vi "receive.vi"(8 "error in (no error)":errorcluster, 11 "ILCCommunications in":refnum<class "ILCCommunications.lvclass">) -> (0 "error out":errorcluster, 3 "ILCCommunications out":refnum<class "ILCCommunications.lvclass">)   [LabVIEW 2016, in "ILCCommunications.lvclass"]
uses:
  ILCCommunications.lvclass
  ILCCommunications.lvclass/ILCCommunications.ctl
  Common_RT_Modbus/DynamicFrameParser/DynamicFrameParser.lvclass
  Common_RT_FPGA/IReadU16FIFO/IReadU16FIFO.lvclass
  Common_RT_Modbus/IModbus/IModbus.lvclass
  Common_RT_HPILC/HPILC/HPILC.lvclass
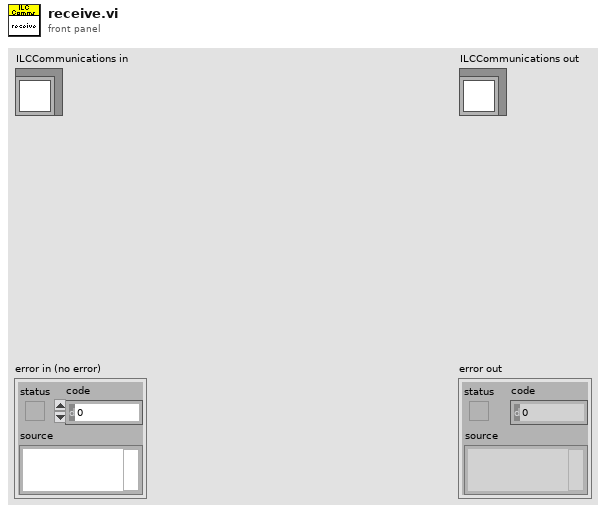
[diagram p1: front panel]
types:
  T1 = typedef "RTModbus.lvlib/RxFrame.ctl" = cluster{"Data":u8[], "Timestamp":u64}
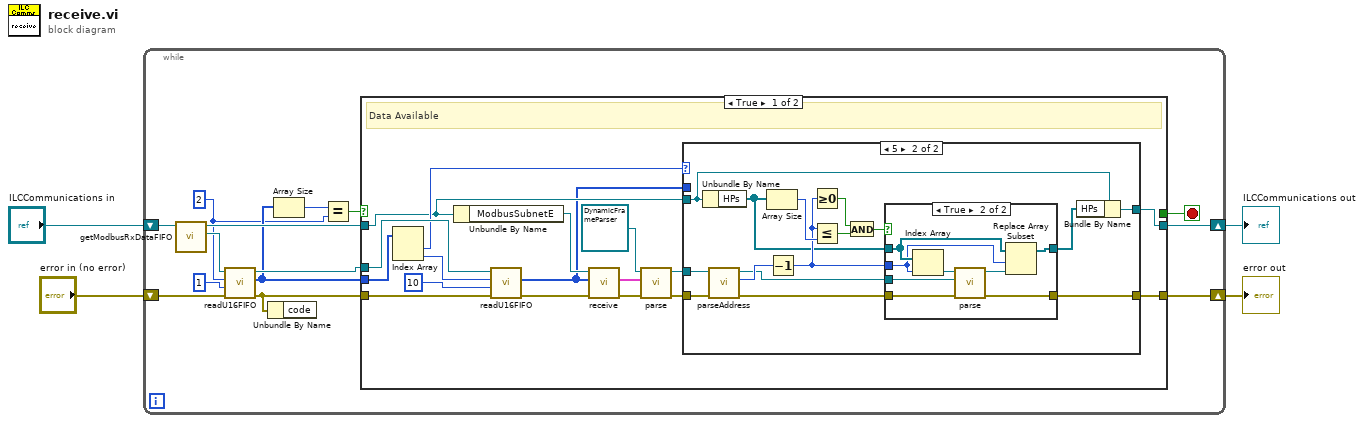
[diagram p0: block diagram]
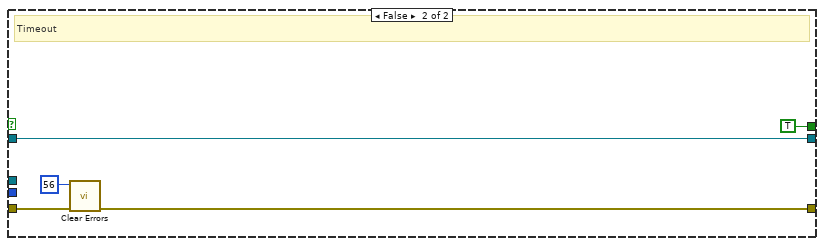
[diagram p4: hidden frame]
diagram:
  n1 = while {
    shift-right: [w13] -> w3
    shift-left: "ILCCommunications in" -> [w18]
    shift-right: [w11] -> w1
    shift-left: "error in (no error)" -> [w12]
    stop <- w9 stop-if-true
    w6 = u32 2 ("NumberOfElements")
    n2 = call "getModbusRxDataFIFO.vi"("ILCCommunications in"=w18) -> ("ModbusRxDataFIFO"=w17:refnum<class "IReadU16FIFO.lvclass">, "ILCCommunications out"=w14:refnum<class "ILCCommunications.lvclass">)  [unwired: 9 in]
    n3 = call-dynamic "readU16FIFO.vi"("error in (no error)"=w12, "Timeout"=1, "NumberOfElements"=w6, "IReadU16FIFO in"=w17) -> ("error out"=w10:errorcluster, "Data"=w8:u16[], "IReadU16FIFO out"=w15:refnum<class "IReadU16FIFO.lvclass">)  [unwired: 4 in, 1 out]
    n4 = Unbundle By Name(w10) -> ()  [unwired: 1 out]
    n5 = Array Size(array=w8) -> (size(s)=w7:i32)
    n6 = Equal?(x=w7, y=w6) -> (x = y?=w5:bool)
    n7 = case shown="True" w5 {
      tunnel: w8 -> [w35 _]
      tunnel: w15 -> [w34 _]
      tunnel: w14 -> [w30 w67]
      tunnel: [w24 w67] -> w13
      tunnel: [w20 w63] -> w11
      tunnel: w10 -> [w19 w64]
      tunnel: [_ TRUE] -> w9
      frame True {
        # "Data Available"
        n8 = Index Array(array=w35) -> (element #1=w31:u16, element #2=w33:u16)  [unwired: 2 in]
        n9 = Unbundle By Name(w30) -> ("ModbusSubnetE"=w29:refnum<class "IModbus.lvclass">)
        n10 = call-dynamic "readU16FIFO.vi"("error in (no error)"=w19, "Timeout"=10, "NumberOfElements"=w33, "IReadU16FIFO in"=w34) -> ("error out"=w23:errorcluster, "Data"=w28:u16[])  [unwired: 4 in, 2 out]
        n11 = call-dynamic "receive.vi"("error in (no error)"=w23, "Data"=w28, "IModbus in"=w29) -> ("error out"=w22:errorcluster, "RxFrame"=w26:T1)  [unwired: 6 in, 1 out]
        n12 = call "parse.vi"("error in (no error)"=w22, "RxFrame"=w26, "FrameParser in"=refnum<class "DynamicFrameParser.lvclass"> refnum ("RTModbus.lvlib:DynamicFrameParser.lvclass")) -> ("error out"=w21:errorcluster, "FrameParser out"=w25:refnum<class "DynamicFrameParser.lvclass">)  [unwired: 7 in]
        n13 = case shown="5" w31 {
          tunnel: w30 -> [w37 w43]
          tunnel: w28 -> [_ _]
          tunnel: w25 -> [_ w47]
          tunnel: [w37 w41] -> w24
          tunnel: w21 -> [w36 w40]
          tunnel: [w36 w38] -> w20
          frame 0, Default {
          }
          frame 5 {
            n14 = Unbundle By Name(w43) -> ("HPs"=w45:refnum<class "HPILC.lvclass">[])
            n15 = call "parseAddress.vi"("error in (no error)"=w40, "FrameParser in"=w47) -> ("error out"=w39:errorcluster, "Address"=w46:u8, "FrameParser out"=w44:refnum<class "DynamicFrameParser.lvclass">)  [unwired: 7 in]
            n16 = Array Size(array=w45) -> (size(s)=w50:i32)
            n17 = Decrement(x=w46) -> (x-1=w48:u8)
            n18 = Greater Or Equal To 0?(x=w48) -> (x >= 0?=w52:bool)
            n19 = Less Or Equal?(x=w48, y=w50) -> (x <= y?=w51:bool)
            n20 = And(x=w52, y=w51) -> (x .and. y?=w49:bool)
            n21 = case shown="True" w49 {
              tunnel: w48 -> [_ w59]
              tunnel: w45 -> [w54 w60]
              tunnel: w44 -> [_ w61]
              tunnel: [w54 w57] -> w42
              tunnel: w39 -> [w53 w56]
              tunnel: [w53 w55] -> w38
              frame False {
              }
              frame True {
                n22 = Index Array(array=w60, index=w59) -> (element=w62:refnum<class "HPILC.lvclass">)
                n23 = call-dynamic "parse.vi"("error in (no error)"=w56, "DynamicFrameParser"=w61, "HPILC in"=w62) -> ("error out"=w55:errorcluster, "HPILC out"=w58:refnum<class "HPILC.lvclass">)  [unwired: 6 in, 1 out]
                n24 = Replace Array Subset(array=w60, new element=w58, index=w59) -> (w57:refnum<class "HPILC.lvclass">[])
              }
            }
            n25 = Bundle By Name(cluster=w43, "HPs"=w42) -> (w41:refnum<class "ILCCommunications.lvclass">)
          }
        }
      }
      frame False {
        # "Timeout"
        n26 = call <vilib>:"Clear Errors.vi"("error in (no error)"=w64, "specific error code to clear (0: all)"=56) -> ("error out"=w63:errorcluster)  [unwired: 4 in, 1 out]
      }
    }
  }
  "error out" <- w1
  "ILCCommunications out" <- w3
